vi "Single Channel FPGA.vi"(4 "Reset by Enc C":bool, 5 "Reset by hand":bool, 6 "DIR":bool, 7 "Period (Ticks)":u32=2000, 8 "STBY":bool, 9 "ENA":bool, 10 "Duty":fxp<+,32,0>, 11 "IO Channels":T1={"PWM In"="Connector1/DIO20", "Direction"="Connector1/DIO20", "ENA"="Connector1/DIO20", "Encoder C"="Connector1/DIO20", "Encoder B"="Connector1/DIO20", "Encoder A"="Connector1/DIO20", "STBY"="Connector1/DIO20"}) -> (2 "JumpBy2Error":i16, 3 "Position":i32)   [LabVIEW 2018, in "jmslib.lvlib"]
uses:
  AppData/Local/Temp/Temp1_StageControl.zip/StageControl/Library/jmslib.lvlib
  <vilib>/eio/EIONode/EIONode.xnode
  <vilib>/rvi/eio/common/nirviEmuTemplateMethod_errors.vi
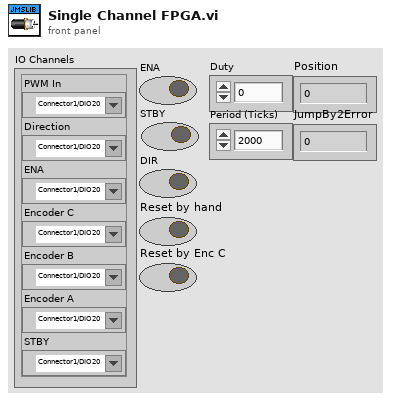
[diagram p1: front panel]
types:
  T1 = cluster{"PWM In":refnum<k21>, "Direction":refnum<k21>, "ENA":refnum<k21>, "Encoder C":refnum<k21>, "Encoder B":refnum<k21>, "Encoder A":refnum<k21>, "STBY":refnum<k21>}
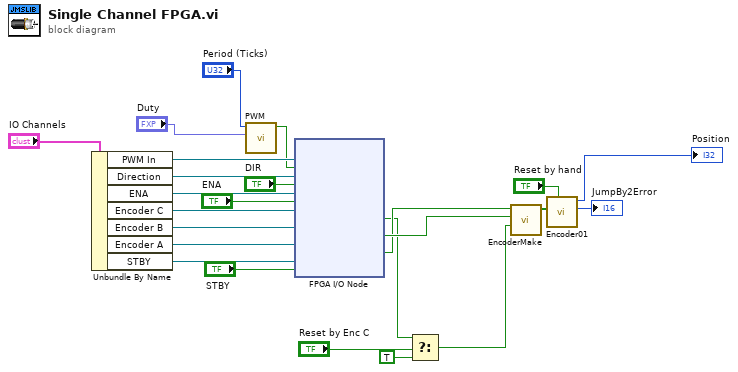
[diagram p0: block diagram]
diagram:
  n1 = Unbundle By Name("IO Channels") -> ("PWM In"=w16:refnum<k21>, "Direction"=w15:refnum<k21>, "ENA"=w14:refnum<k21>, "Encoder C"=w12:refnum<k21>, "Encoder B"=w11:refnum<k21>, "Encoder A"=w10:refnum<k21>, "STBY"=w9:refnum<k21>)
  n2 = call "PWM.vi"("Duty Cycle"="Duty", "Period (Ticks)"="Period (Ticks)") -> ("PWM Out"=w13:bool)  [unwired: 8 in, 1 out]
  n3 = xnode "FPGA I/O Node"("I/O Item"=w13, "FPGA I/O In"=w16, "I/O Item"="DIR", "FPGA I/O In"=w15, "I/O Item"="ENA", "FPGA I/O In"=w14, "FPGA I/O In"=w12, "FPGA I/O In"=w11, "FPGA I/O In"=w10, "I/O Item"="STBY", "FPGA I/O In"=w9) -> ("I/O Item"=w2:bool, "I/O Item"=w21:bool, "I/O Item"=w20:bool)  [unwired: 7 out]
  n4 = Select(t=w2, s="Reset by Enc C", f=TRUE ("C")) -> (s? t:f=w3:bool)
  n5 = call "EncoderMake.vi"("C"=w3, "B"=w21, "A"=w20) -> ("Encoder Array"=w19:bool[])  [unwired: 8 in]
  n6 = call "Encoder01.vi"("ForceReset"="Reset by hand", "Encoder Array"=w19) -> ("JumpBy2Error"=→"JumpBy2Error":i16, "Position"=→"Position":i32)  [unwired: 6 in, 2 out]
